vi "Get APU SubTests.vi"(11 "Controller (Host) Data in":T1) -> (3 "SubTests Array out":string[](array[string]))   [LabVIEW 2018]
uses:
  <userlib>/_OpenG.lib/array/array.llb/Filter 1D Array with Scalar (String)__ogtk.vi
  Public Controls/APU Select.ctl
  Controller (Host).lvlib
  Private Controls/State.ctl
  Private Controls/Controller (Host) Data.ctl
  Top Level/Shared Controls/APU Setup File.ctl
  Public Controls/Test Information.ctl
  Top Level/Shared Controls/Calculated Data.ctl
panel:
  # "Test Information:"
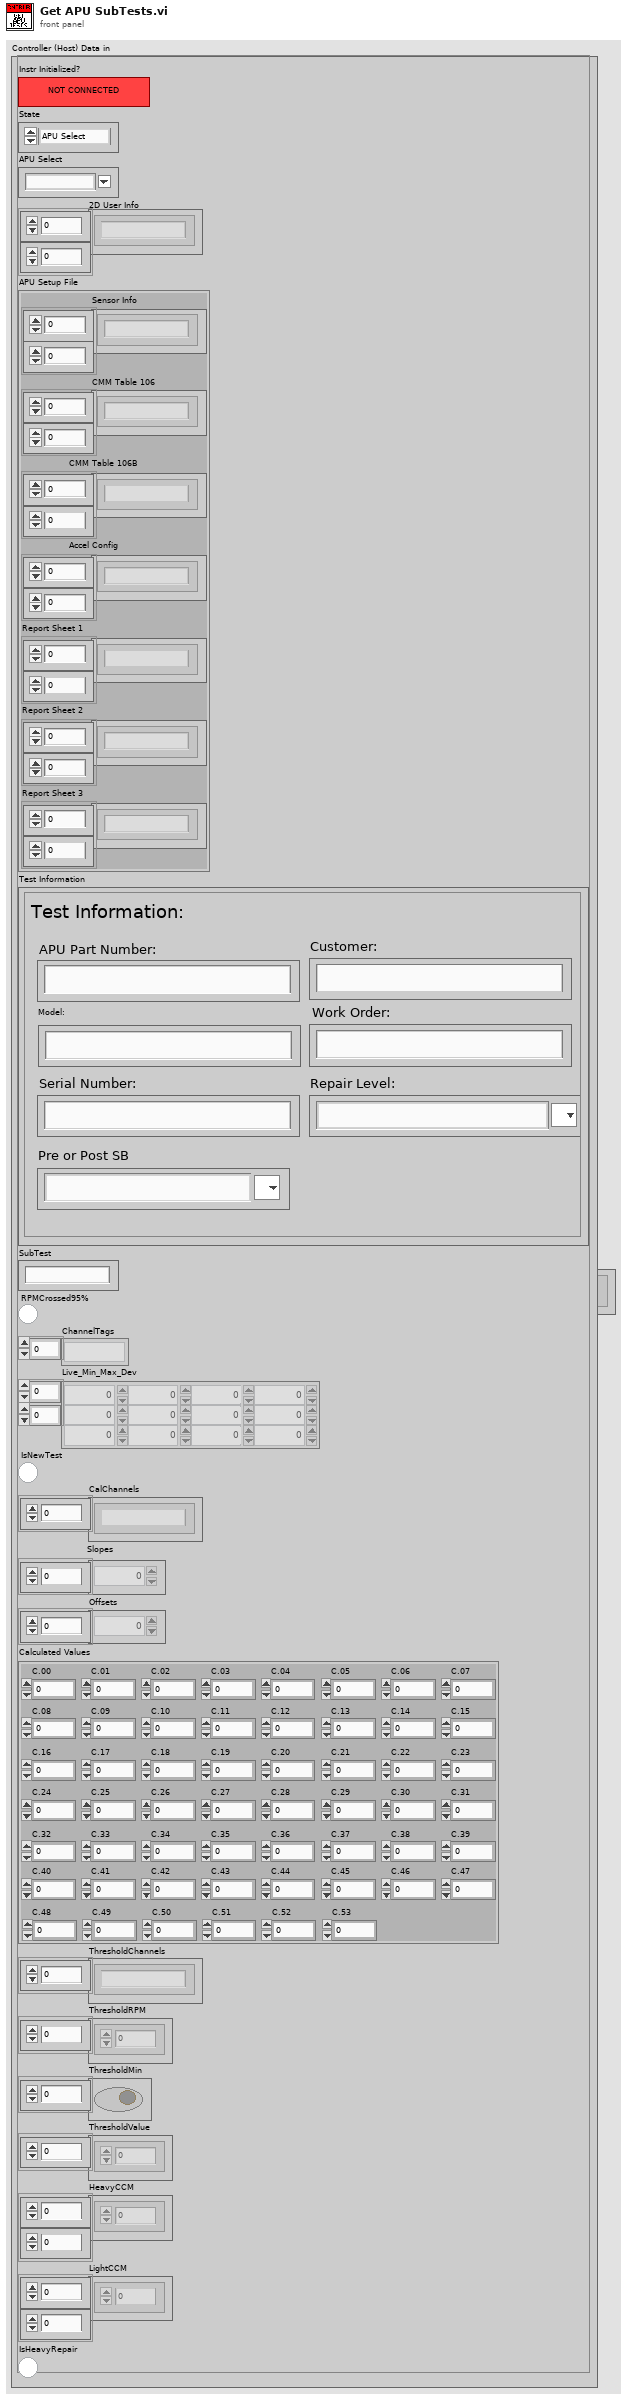
[diagram p1: front panel]
types:
  T1 = typedef "Controller (Host).lvlib/Controller (Host) Data.ctl" = cluster{"Instr Initialized?":bool, "State":T2, "APU Select":T3, "2D User Info":string[][], "APU Setup File":T4, "Test Information":T5, "SubTest":string, "RPMCrossed95%":bool, "ChannelTags":string[], "Live_Min_Max_Dev":dbl[][], "IsNewTest":bool, "CalChannels":string[], "Slopes":dbl[], "Offsets":dbl[], "Calculated Values":T6, "ThresholdChannels":string[], "ThresholdRPM":dbl[], "ThresholdMin":bool[], "ThresholdValue":dbl[], "HeavyCCM":dbl[][], "LightCCM":dbl[][], "IsHeavyRepair":bool}
  T2 = typedef "Controller (Host).lvlib/State.ctl" = enum16{"APU Select", "Operation Select", "SubTests Select", "Calibration", "Testing", "Exit"}
  T3 = typedef "Controller (Host).lvlib/APU Select.ctl" = string
  T4 = typedef "APU Setup File.ctl" = cluster{"Sensor Info":string[][], "CMM Table 106":string[][], "CMM Table 106B ":string[][], "Accel Config":string[][], "Report Sheet 1":string[][], "Report Sheet 2":string[][], "Report Sheet 3":string[][]}
  T5 = typedef "Controller (Host).lvlib/Test Information.ctl" = cluster{"APU Part Number:":string, "Model:":string, "Serial Number:":string, "Customer:":string, "Work Order:":string, "Repair Level:":string, "Pre or Post SB":string}
  T6 = typedef "Calculated Data.ctl" = cluster{"C.00":dbl, "C.01":dbl, "C.02":dbl, "C.03":dbl, "C.04":dbl, "C.05":dbl, "C.06":dbl, "C.07":dbl, "C.08":dbl, "C.09":dbl, "C.10":dbl, "C.11":dbl, "C.12":dbl, "C.13":dbl, "C.14":dbl, "C.15":dbl, "C.16":dbl, "C.17":dbl, "C.18":dbl, "C.19":dbl, "C.20":dbl, "C.21":dbl, "C.22":dbl, "C.23":dbl, "C.24":dbl, "C.25":dbl, "C.26":dbl, "C.27":dbl, "C.28":dbl, "C.29":dbl, "C.30":dbl, "C.31":dbl, "C.32":dbl, "C.33":dbl, "C.34":dbl, "C.35":dbl, "C.36":dbl, "C.37":dbl, "C.38":dbl, "C.39":dbl, "C.40":dbl, "C.41":dbl, "C.42":dbl, "C.43":dbl, "C.44":dbl, "C.45":dbl, "C.46":dbl, "C.47":dbl, "C.48":dbl, "C.49":dbl, "C.50":dbl, "C.51":dbl, "C.52":dbl, "C.53":dbl}
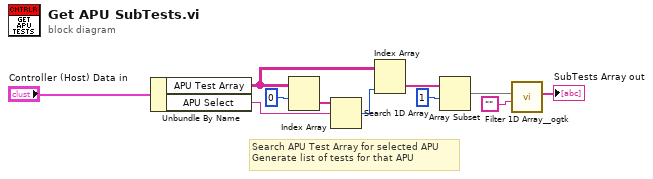
[diagram p0: block diagram]
diagram:
  # "Search APU Test Array for selected APU\nGenerate list of tests for that APU"
  n1 = Unbundle By Name("Controller (Host) Data in") -> ("APU Test Array"=w5:string[][], "APU Select"=w6:T3)
  n2 = Index Array(array=w5, index (row)=0) -> (element=w7:string[])  [unwired: 1 in]
  n3 = Search 1D Array(1D array=w7, element=w6) -> (index of element=w4:i32)  [unwired: 1 in]
  n4 = Index Array(array=w5, index (col)=w4) -> (element=w11:string[])  [unwired: 1 in]
  n5 = Array Subset(array=w11, index=1) -> (w3:string[])  [unwired: 1 in]
  n6 = call-poly <userlib>:"Filter 1D Array__ogtk.vi"("items to filter"="", "array"=w3) -> ("filtered array"=→"SubTests Array out":string[])  [unwired: 4 in, 1 out]
